vi "Disconnect.vi"(8 "error in":errorcluster, 11 "Hitronics in":refnum<class "Hitronics.lvclass">) -> (0 "error out":errorcluster, 3 "Hitronics out":refnum<class "Hitronics.lvclass">)   [LabVIEW 2018, in "Hitronics.lvlib" / "Hitronics.lvclass"]
doc: "Close VISA resource session"
uses:
  Hitronics.lvclass
  PPLs/Laser/Parent/Laser.lvlibp/Laser.lvclass
  C:/AME Test Engineering/LabVIEW/PPLs/Laser/Parent/Laser.lvlibp/Laser.lvclass
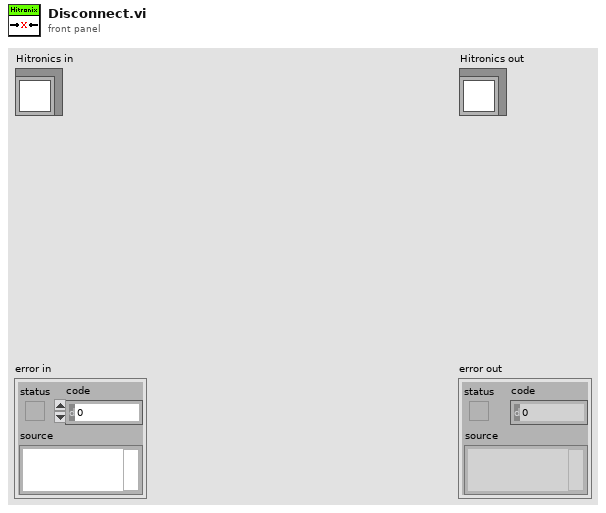
[diagram p1: front panel]
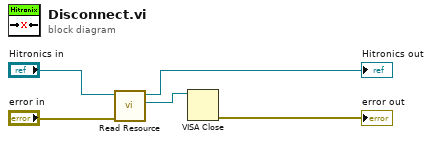
[diagram p0: block diagram]
diagram:
  n1 = call "Read Resource.vi"("error in (no error)"="error in", "Laser in"="Hitronics in") -> ("Resource"=w3:refnum<visa-resource-name>, "Laser out"=→"Hitronics out":refnum<class "Hitronics.lvclass">)  [unwired: 7 in, 1 out]
  n2 = VISA Close(VISA resource name=w3) -> (error out=→"error out":errorcluster)  [unwired: 1 in]
